vi "Write.vi"(8 "error in (no error)":errorcluster, 10 "Data to Write":string, 11 "IConnection in":refnum<class "IConnection.lvclass">) -> (0 "error out":errorcluster, 3 "IConnection out":refnum<class "IConnection.lvclass">)   [LabVIEW 2019, in "Connection Reference.lvlib" / "IConnection.lvclass"]
uses:
  <vilib>/gpm_packages/@cs/Network-interface/Source/Connection Reference/IConnection/IConnection.lvclass
  <vilib>/ErrorRing/Error Ring.xnode
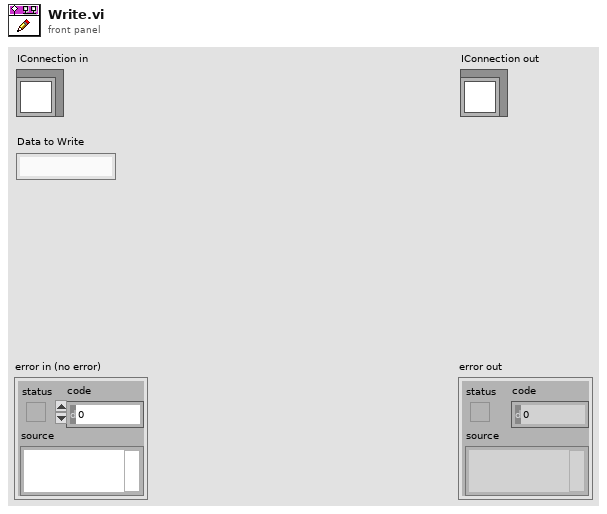
[diagram p1: front panel]
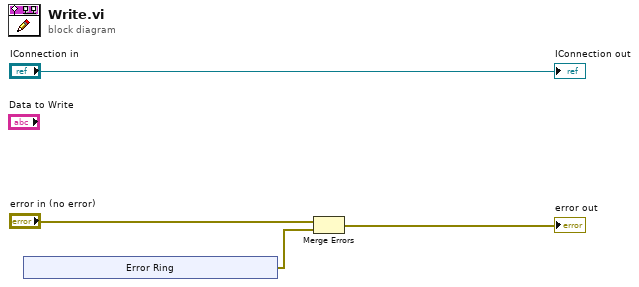
[diagram p0: block diagram]
diagram:
  n1 = xnode "Error Ring"() -> ("error out"=w1:errorcluster)
  n2 = Merge Errors("error in (no error)", w1) -> (→"error out":errorcluster)
  "IConnection out" <- "IConnection in"
